vi "ThreeIncoming_Triggered.vi"() -> ()   [LabVIEW 2019]
uses:
  <vilib>/rvi/DataTransferAndStorage/Container/XNode/niFpgaContainer.xnode
  <vilib>/rvi/interface/RandomDataEmulation/nirviRandomDataFpgaReadWriteTemplate.vi
panel:
  in  "Trigger Medium":bool
  in  "Trigger Slow":bool
  out "Boolean 2":bool=TRUE
  out "Fast timeout":bool
  out "Med timeout":bool
  out "Slow timeout":bool
  in  "I16":i16
  in  "I8":i8
  in  "I64":i64
  in  "I32":i32
  in  "U16":u16
  in  "U8":u8
  in  "U64":u64
  in  "U32":u32
  in  "SGL":sgl
  in  "Boolean":bool
  out "I16 out":i16
  out "I8 out":i8
  out "I64 out":i64
  out "I32 out":i32
  out "U16 out":u16
  out "U8 out":u8
  out "U64 out":u64
  out "U32 out":u32
  out "SGL out":sgl
  out "Boolean out":bool
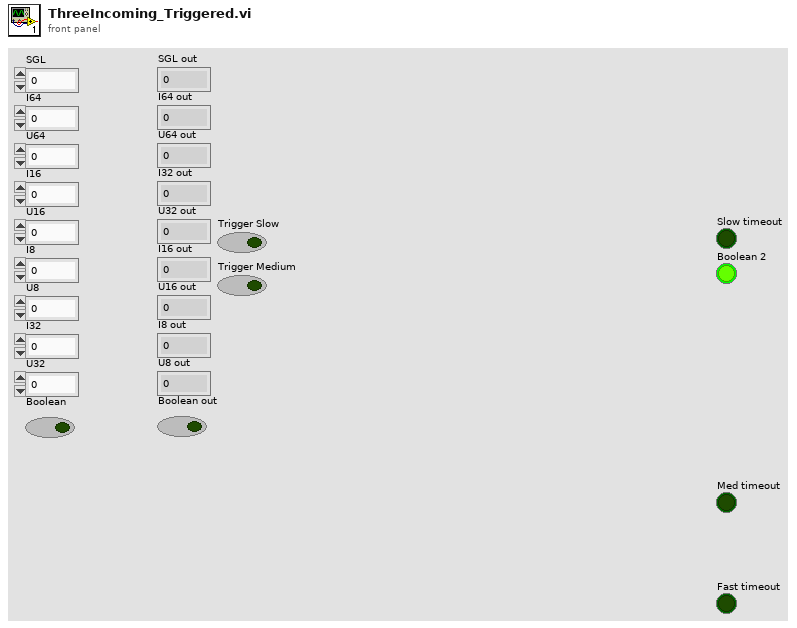
[diagram p1: front panel]
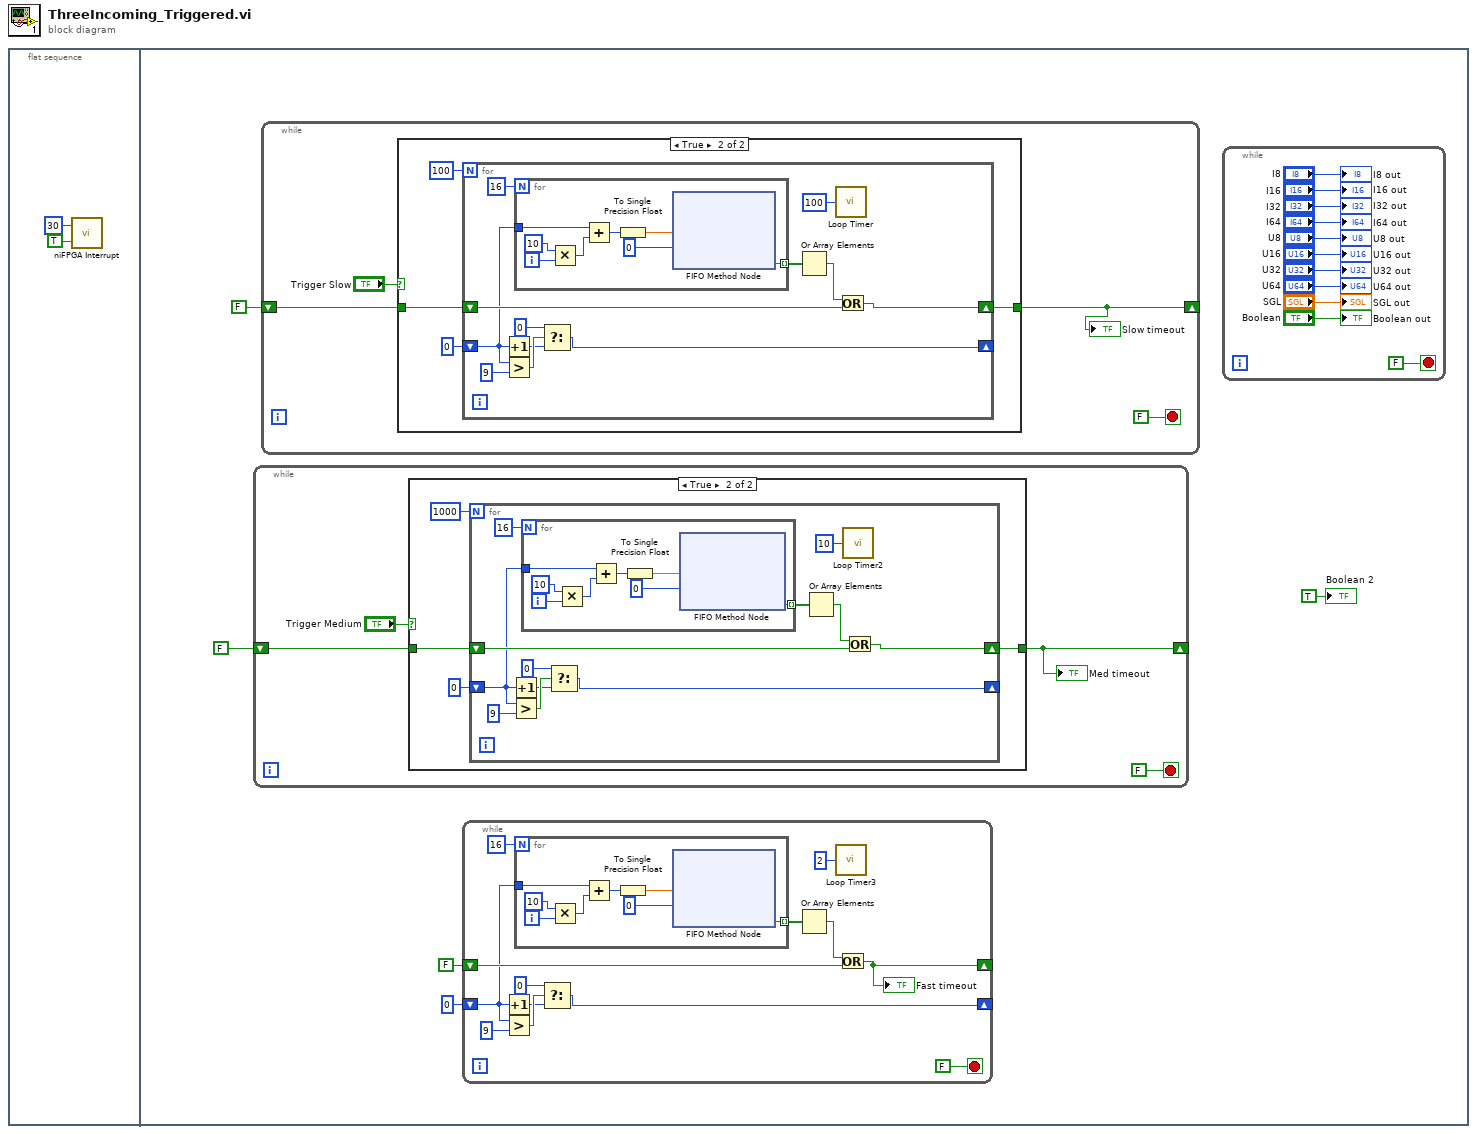
[diagram p0: block diagram]
diagram:
  n1 = flat-sequence {
    frame #0 {
      n2 = call <vilib>:"niFPGA Interrupt.vi"("Wait Until Cleared (F)"=TRUE, "IRQ Number (0)"=u8 30) -> ()  [unwired: 1 in]
    }
    frame #1 {
      n3 = while {
        shift-right: [w30] -> _
        shift-left: FALSE -> [w29]
        stop <- FALSE stop-if-true
        n4 = case shown="True" "Trigger Medium" {
          tunnel: [w33 w35] -> w30
          tunnel: w29 -> [w33 w34]
          frame False {
          }
          frame True {
            n5 = for {
              N: 1000 -> [_]
              shift-right: [w44] -> _
              shift-left: 0 ("t") -> [w38]
              shift-right: [w39] -> w35
              shift-left: w34 -> [w40]
              n6 = Increment(x=w38) -> (x+1=w43:i32)
              n7 = Greater?(x=w38, y=9) -> (0:w48:bool)
              n8 = for {
                N: 16 -> [_]
                tunnel: w38 -> [w57]
                tunnel: [w50] -> w42 mode=indexing
                i -> [w56]
                n9 = Multiply(x=10, y=w56) -> (x*y=w54:i32)
                n10 = Add(x=w57, y=w54) -> (x+y=w53:i32)
                n11 = To Single Precision Float(number=w53) -> (single precision float=w52:sgl)
                n12 = xnode ("FIFO Method Node")("Element"=w52, "Timeout"=0) -> ("Timed Out?"=w50:bool)  [unwired: 1 in, 1 out]
              }
              n13 = Select(t=0, s=w48, f=w43) -> (s? t:f=w44:i32)
              n14 = Or Array Elements(Boolean array=w42) -> (logical OR=w41:bool)
              n15 = call "Loop Timer2"("Count(uSec)"=u32 10) -> ()  [unwired: 1 out]
              n16 = Or(x=w41, y=w40) -> (x .or. y?=w39:bool)
            }
          }
        }
        "Med timeout" <- w30
      }
      n17 = while {
        shift-right: [w59] -> _
        shift-left: FALSE -> [w58]
        stop <- FALSE stop-if-true
        n18 = case shown="True" "Trigger Slow" {
          tunnel: [w62 w64] -> w59
          tunnel: w58 -> [w62 w63]
          frame False {
          }
          frame True {
            n19 = for {
              N: 100 -> [_]
              shift-right: [w73] -> _
              shift-left: 0 ("t") -> [w67]
              shift-right: [w68] -> w64
              shift-left: w63 -> [w69]
              n20 = Increment(x=w67) -> (x+1=w72:i32)
              n21 = Greater?(x=w67, y=9) -> (0:w77:bool)
              n22 = for {
                N: 16 -> [_]
                tunnel: w67 -> [w86]
                tunnel: [w79] -> w71 mode=indexing
                i -> [w85]
                n23 = Multiply(x=10, y=w85) -> (x*y=w83:i32)
                n24 = Add(x=w86, y=w83) -> (x+y=w82:i32)
                n25 = To Single Precision Float(number=w82) -> (single precision float=w81:sgl)
                n26 = xnode ("FIFO Method Node")("Element"=w81, "Timeout"=0) -> ("Timed Out?"=w79:bool)  [unwired: 1 in, 1 out]
              }
              n27 = Select(t=0, s=w77, f=w72) -> (s? t:f=w73:i32)
              n28 = Or Array Elements(Boolean array=w71) -> (logical OR=w70:bool)
              n29 = call "Loop Timer"("Count(uSec)"=u32 100) -> ()  [unwired: 1 out]
              n30 = Or(x=w70, y=w69) -> (x .or. y?=w68:bool)
            }
          }
        }
        "Slow timeout" <- w59
      }
      n31 = while {
        shift-right: [w15] -> _
        shift-left: 0 ("t") -> [w9]
        shift-right: [w10] -> _
        shift-left: FALSE -> [w11]
        stop <- FALSE stop-if-true
        n32 = Increment(x=w9) -> (x+1=w14:i32)
        n33 = Greater?(x=w9, y=9) -> (0:w19:bool)
        n34 = for {
          N: 16 -> [_]
          tunnel: w9 -> [w28]
          tunnel: [w21] -> w13 mode=indexing
          i -> [w27]
          n35 = Multiply(x=10, y=w27) -> (x*y=w25:i32)
          n36 = Add(x=w28, y=w25) -> (x+y=w24:i32)
          n37 = To Single Precision Float(number=w24) -> (single precision float=w23:sgl)
          n38 = xnode ("FIFO Method Node")("Element"=w23, "Timeout"=0) -> ("Timed Out?"=w21:bool)  [unwired: 1 in, 1 out]
        }
        n39 = Select(t=0, s=w19, f=w14) -> (s? t:f=w15:i32)
        n40 = Or Array Elements(Boolean array=w13) -> (logical OR=w12:bool)
        n41 = call "Loop Timer3"("Count(uSec)"=u32 2) -> ()  [unwired: 1 out]
        n42 = Or(x=w12, y=w11) -> (x .or. y?=w10:bool)
        "Fast timeout" <- w10
      }
      n43 = while {
        stop <- FALSE stop-if-true
        "I16 out" <- "I16"
        "I8 out" <- "I8"
        "I64 out" <- "I64"
        "I32 out" <- "I32"
        "U16 out" <- "U16"
        "U8 out" <- "U8"
        "U64 out" <- "U64"
        "U32 out" <- "U32"
        "SGL out" <- "SGL"
        "Boolean out" <- "Boolean"
      }
      "Boolean 2" <- TRUE
    }
  }
